vi "AfterPage2_ScriptModel.vi"(10 "MetaDataObj":refnum<class "MetaDataObj.lvclass">, 11 "User Project":refnum<vi>) -> ()   [LabVIEW 2014, in "NIVS_ScriptedModuleTemplate_MetaDataObj.lvclass"]
uses:
  NIVS_ScriptedModuleTemplate_MetaDataObj.lvclass
  <resource>/dialog/NewProjectWizard/MetaDataObj/MetaDataObj.lvclass
  <resource>/dialog/NewProjectWizard/MetaDataObj/MetaDataObj.lvclass/MetaDataObj.ctl
  <resource>/dialog/NewProjectWizard/MetaDataObj/Accessors/Read Project Destination Path.vi
  <vilib>/Utility/EditLVProj/Edit LVProj.lvlib
  <resource>/dialog/NewProjectWizard/Project Copying/NI_NPW_Project Copying.lvlib
panel:
  out "error out":errorcluster
  # "Make a copy of this template to implement your own AfterPage2NoUI scripting VI for your custom template/sample project."
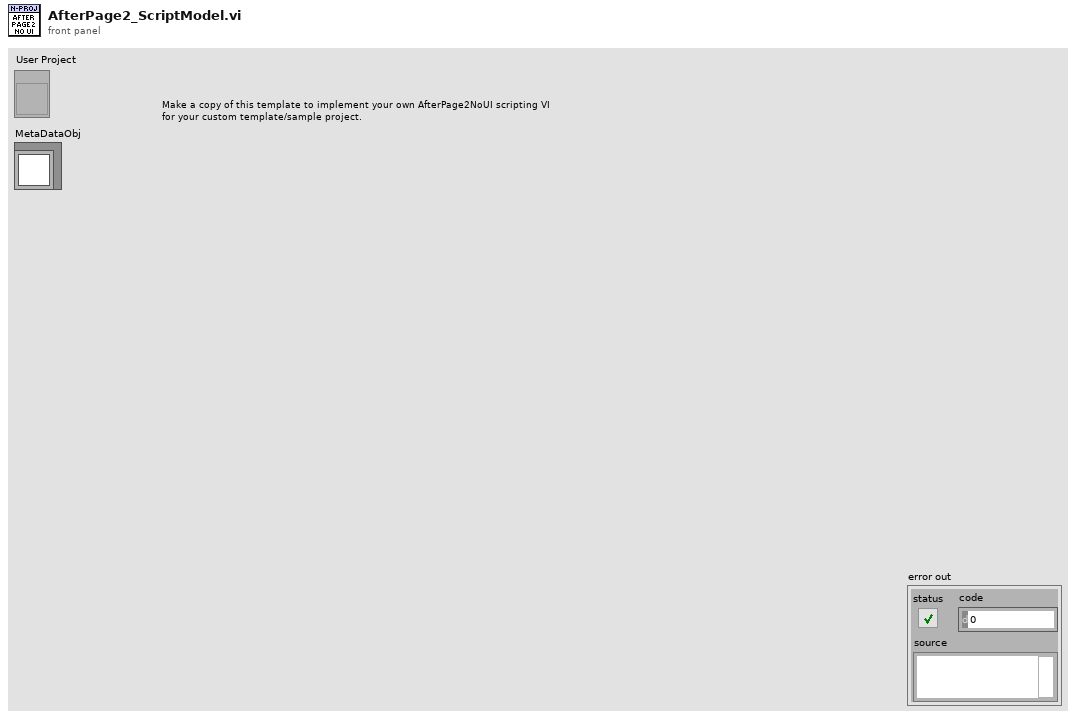
[diagram p1: front panel]
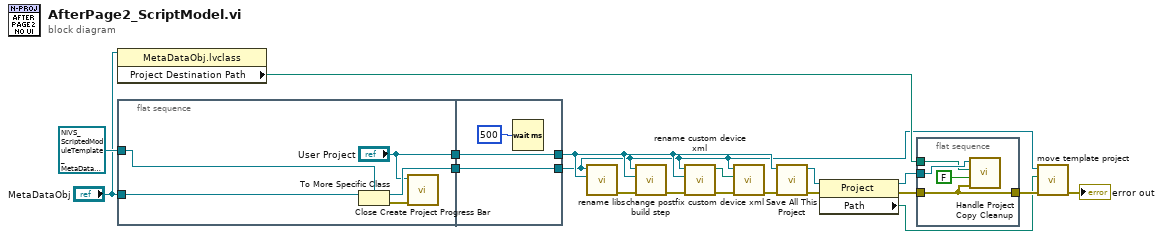
[diagram p0: block diagram]
diagram:
  n1 = property class="MetaDataObj.lvclass"(reference="MetaDataObj") -> ("Project Destination Path"=w11:path)  [unwired: 1 in, 2 out]
  n2 = flat-sequence {
    tunnel: refnum<class "NIVS_ScriptedModuleTemplate_MetaDataObj.lvclass"> refnum ("NIVS_CDW_MetaDataObj.lvclass") -> [w24]
    tunnel: "MetaDataObj" -> [w22]
    tunnel: [w23] -> w9
    tunnel: ["User Project"] -> w8
    tunnel: [w26] -> w10
    tunnel: [w27] -> w1
    tunnel: w9 -> [w27]
    tunnel: w8 -> [w26]
    frame #0 {
      n3 = To More Specific Class(target class=w24, reference=w22) -> (specific class reference=w23:refnum<class "NIVS_ScriptedModuleTemplate_MetaDataObj.lvclass">, error out=w21:errorcluster)  [unwired: 1 in]
      n4 = call <resource>:"Close Create Project Progress Bar.vi"("error in (no error)"=w21, "Project"="User Project") -> ()  [unwired: 8 in, 2 out]
    }
    frame #1 {
      n5 = Wait (ms)(milliseconds to wait=u32 500) -> ()  [unwired: 1 out]
    }
  }
  n6 = call "rename libs.vi"("User Project"=w10, "NIVS_CDW_MetaDataObj in"=w1) -> ("error out"=w17:errorcluster)  [unwired: 9 in]
  n7 = call "change post build step.vi"("error in (no error)"=w17, "User Project"=w10, "NIVS_CDW_MetaDataObj in"=w1) -> ("error out"=w18:errorcluster)  [unwired: 8 in]
  n8 = call "rename custom device xml.vi"("error in (no error)"=w18, "User Project"=w10, "NIVS_CDW_MetaDataObj in"=w1) -> ("error out"=w16:errorcluster, "new xml path"=w15:path)  [unwired: 7 in]
  n9 = call "fix custom device xml.vi"("error in (no error)"=w16, "new xml path"=w15, "NIVS_CDW_MetaDataObj in"=w1) -> ("error out"=w14:errorcluster)  [unwired: 8 in]
  n10 = call <vilib>:"Save All This Project.vi"("error in (no error)"=w14, "Project in"=w10) -> ("error out"=w13:errorcluster, "Project out"=w5:refnum<vi>)  [unwired: 8 in]
  n11 = property class="Project"(reference=w5, error in=w13) -> (reference out=w4:refnum<vi>, error out=w6:errorcluster, "Path"=w3:path)
  n12 = flat-sequence {
    tunnel: w6 -> [w28]
    tunnel: w4 -> [w31]
    tunnel: w11 -> [w30]
    tunnel: [w28] -> w7
    frame #0 {
      n13 = call <resource>:"Handle Project Copy Cleanup.vi"("error in (no error)"=w28, "More Scripting?"=FALSE, "Target Path"=w30, "Project in"=w31) -> ()  [unwired: 8 in]
    }
  }
  n14 = call "move template project.vi"("error in (no error)"=w7, "Path"=w3, "NIVS_ScriptedModuleTemplate_MetaDataObj in"=w1) -> ("error out"=→"error out":errorcluster)  [unwired: 8 in]
